vi "Curtin_ChannelType.vi"(2 "Channel 1 [Right]":u16(ring)=2 items=["Accelerometer", "Accel(Speed)", "Microphone", "Velocimeter", "Piezo"], 3 "Mic":waveform(dbl)(graph)) -> (1 "Mic out":waveform(dbl)(graph))   [LabVIEW 2022 SP3]
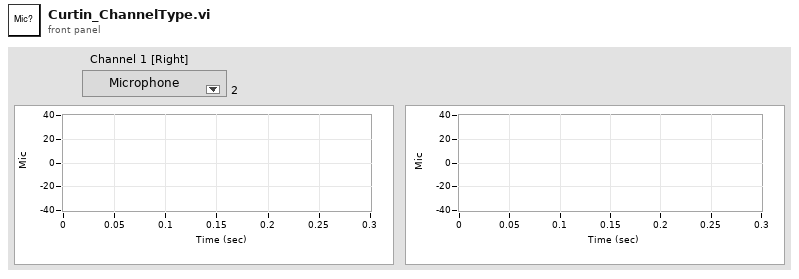
[diagram p1: front panel]
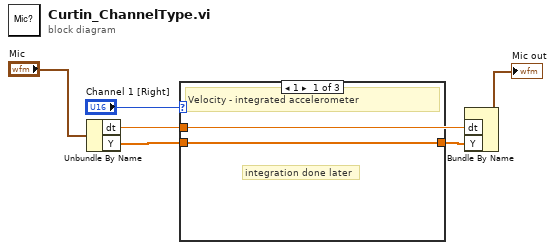
[diagram p0: block diagram]
diagram:
  n1 = Unbundle By Name("Mic") -> ("dt"=w1:dbl, "Y"=w3:dbl[])
  n2 = case shown="1" "Channel 1 [Right]" {
    tunnel: [w7 w8 w9] -> w4
    tunnel: w3 -> [w7 w8 w9]
    tunnel: w1 -> [_ _ _]
    frame 1 {
      # "integration done later"
      # "Velocity - integrated accelerometer"
    }
    frame 0, 2..4 {
      # "Accelerometer, Microphone, Vibrometer"
    }
    frame Default {
    }
  }
  n3 = Bundle By Name("dt"=w1, "Y"=w4) -> (→"Mic out":waveform(dbl))  [unwired: 1 in]
